vi "util.DelimitedStringFromArray.vi"(9 "delimiter (Comma)":string=",", 10 "params array in":string[](array[string])) -> (2 "delimited string out":string)   [LabVIEW 2024]
uses:
  <vilib>/Utility/error.llb/Trim Whitespace One-Sided.vi
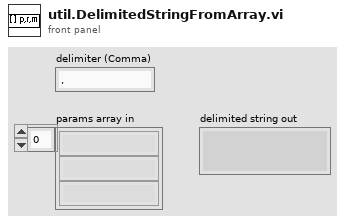
[diagram p1: front panel]
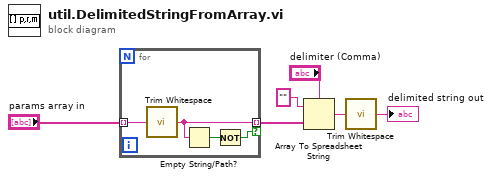
[diagram p0: block diagram]
diagram:
  n1 = for {
    tunnel: "params array in" -> [w10] mode=indexing
    tunnel: [w7] -> w1 mode=indexing if=w8
    n2 = call <vilib>:"Trim Whitespace.vi"("string"=w10) -> ("trimmed string"=w7:string)  [unwired: 1 in]
    n3 = Empty String/Path?(string/path=w7) -> (empty?=w9:bool)
    n4 = Not(x=w9) -> (.not. x?=w8:bool)
  }
  n5 = Array To Spreadsheet String(delimiter (Tab)="delimiter (Comma)", array=w1, 3:"" ("format string")) -> (spreadsheet string=w4:string)
  n6 = call <vilib>:"Trim Whitespace.vi"("string"=w4) -> ("trimmed string"=→"delimited string out":string)  [unwired: 1 in]
